vi "start.vi"(8 "error in (no error)":errorcluster, 11 "EncoderReader in":refnum<class "EncoderReader.lvclass">) -> (0 "error out":errorcluster, 3 "EncoderReader out":refnum<class "EncoderReader.lvclass">)   [LabVIEW 2013, in "EncoderReader.lvclass"]
uses:
  EncoderReader.lvclass
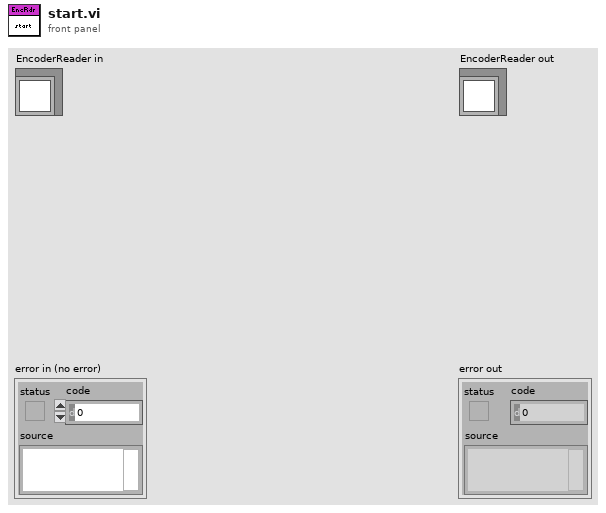
[diagram p1: front panel]
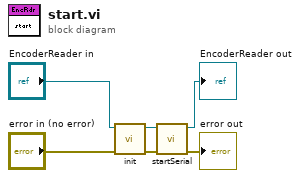
[diagram p0: block diagram]
diagram:
  n1 = call "init.vi"("error in (no error)"="error in (no error)", "EncoderReader in"="EncoderReader in") -> ("error out"=w3:errorcluster, "EncoderReader out"=w6:refnum<class "EncoderReader.lvclass">)  [unwired: 8 in]
  n2 = call "startSerial.vi"("error in (no error)"=w3, "EncoderReader in"=w6) -> ("error out"=→"error out":errorcluster, "EncoderReader out"=→"EncoderReader out":refnum<class "EncoderReader.lvclass">)  [unwired: 8 in]
